vi "keep val.vi"(4 "in":bool) -> (1 "out":bool)   [LabVIEW 2012]
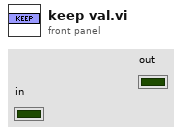
[diagram p1: front panel]
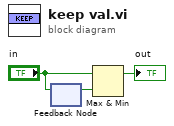
[diagram p0: block diagram]
diagram:
  n1 = feedback #1() -> (w3:bool)  [unwired: 1 in]
  n2 = feedback-in #1("in") -> ()
  n3 = Max & Min(x="in", y=w3) -> (max(x,y)=→"out":bool)  [unwired: 1 out]
